vi "Calibrate Ticks 2 Timeout (uSMC).vi"(1 "Timeouts (Ticks)":u16) -> (0 "Timeout (ms)":u16)   [LabVIEW 2010, in "SignalWriterMH110203USBStepperMotor.lvclass"]
uses:
  SignalWriterMH110203USBStepperMotor.lvclass
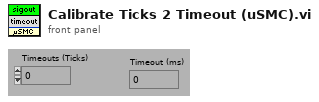
[diagram p1: front panel]
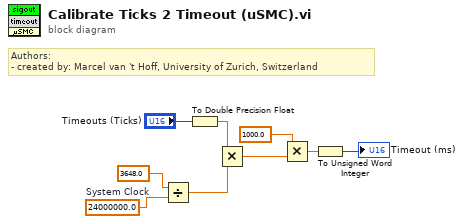
[diagram p0: block diagram]
diagram:
  w9 = 24000000.0  # System Clock
  # "Authors: \n- created by: Marcel van 't Hoff, University of Zurich, Switzerland"
  n1 = Divide(x=3648.0 ("y"), y=w9) -> (x/y=w7:dbl)
  n2 = To Double Precision Float(number="Timeouts (Ticks)") -> (double precision float=w4:dbl)
  n3 = Multiply(x=w4, y=w7) -> (x*y=w5:dbl)
  n4 = Multiply(x=1000.0, y=w5) -> (x*y=w3:dbl)
  n5 = To Unsigned Word Integer(number=w3) -> (unsigned 16bit integer=→"Timeout (ms)":u16)
